vi "lvssh2_session_callback_send_handler_32.vi"(9 "lvssh2_session_callback_send":refnum<vi>, 10 "Stop Event Ref":refnum<user-event>, 11 "User Event Ref":refnum<user-event>) -> ()   [LabVIEW 2017, in "libssh2.lvlib"]
uses:
  libssh2.lvlib
  lvssh2_session_callback_send_function_input_args_32.ctl
  lvssh2_extensions_64.dll
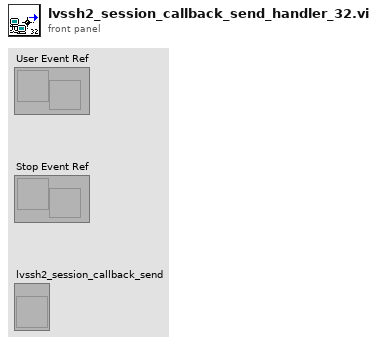
[diagram p1: front panel]
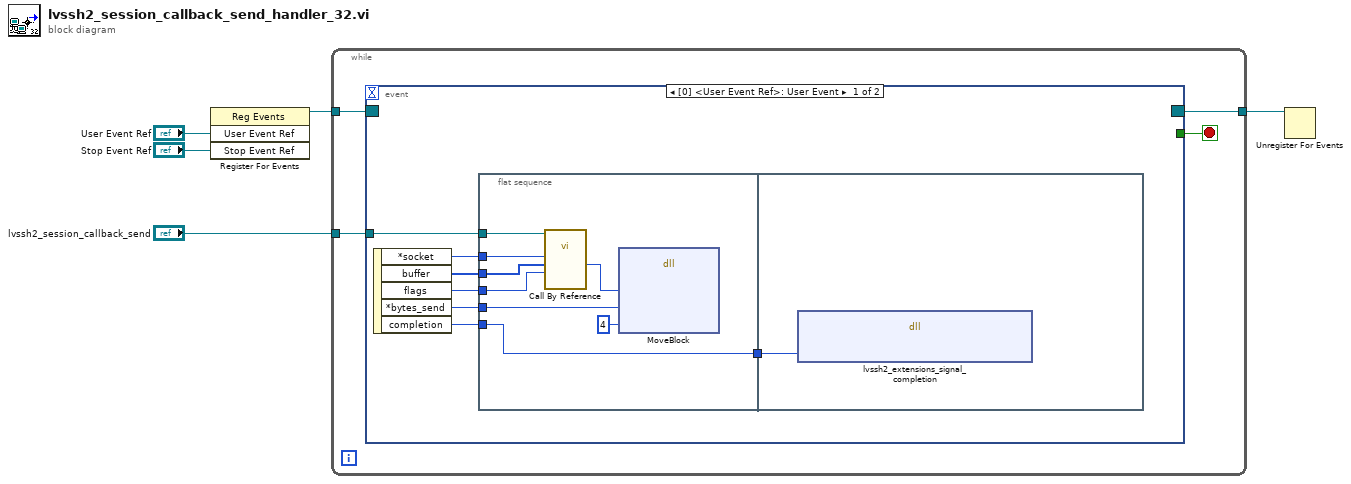
[diagram p0: block diagram]
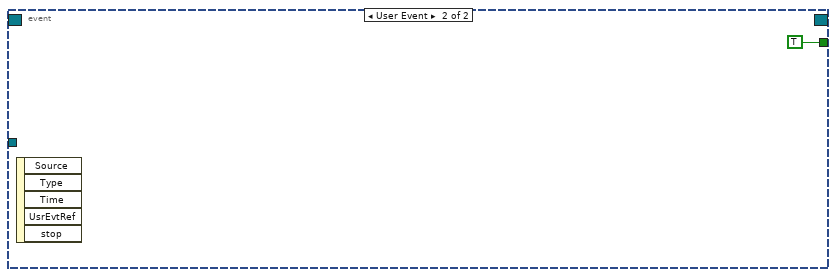
[diagram p2: hidden frame]
diagram:
  n1 = register-events("User Event Ref", "Stop Event Ref") -> (reference out=w4:refnum<event-registration>)  [unwired: 2 in, 1 out]
  n2 = while {
    tunnel: "lvssh2_session_callback_send" -> [w9]
    tunnel: w4 -> [w8]
    tunnel: [w7] -> w1
    stop <- w6 stop-if-true
    n3 = event shown="[0] <User Event Ref>: User Event" {
      selector: w8 -> [_ _]
      dyn-events: [_ _] -> w7
      timeout: _ -> [_ _]
      tunnel: w9 -> [w15 _]
      tunnel: [_ TRUE] -> w6
      event User Event {
        n4 = event-data() -> ("*socket"=w14:u32, "buffer"=w13:u8[], "flags"=w12:i32, "*bytes_send"=w11:u32, "completion"=w10:u32)  [unwired: 1 in]
        n5 = flat-sequence {
          tunnel: w15 -> [w24]
          tunnel: w14 -> [w23]
          tunnel: w12 -> [w22]
          tunnel: w13 -> [w21]
          tunnel: w11 -> [w19]
          tunnel: [w17] -> w16
          tunnel: w10 -> [w17]
          tunnel: w16 -> [w25]
          frame #0 {
            n6 = call-by-ref "?"(reference=w24, "flags"=w22, "buffer"=w21, "socket"=w23) -> ("bytes send"=w18:i64)  [unwired: 8 in, 3 out]
            n7 = dll-call lib="LabVIEW" fn="MoveBlock"("ps"=w18, "pd"=w19, "size"=u64 4) -> ()  [unwired: 7 in, 2 out]
          }
          frame #1 {
            n8 = dll-call lib="C:/Users/Pascal/Projects/Home/lvssh2/libssh2/lvssh2_extensions**.*" fn="lvssh2_extensions_signal_completion"("completion"=w25) -> ()  [unwired: 5 in, 2 out]
          }
        }
      }
      event User Event {
        n9 = event-data() -> ()  [unwired: 1 in, 5 out]
      }
    }
  }
  n10 = Unregister For Events(event registration refnum=w1) -> ()  [unwired: 1 in, 1 out]
